vi "Lab Panel V4.83.vi"() -> ()   [LabVIEW 2013] (continued)
                    n2337 = Bundle("FAIL LAB02-2"=w3939, "SIG LAB02-2"=w3949, "TEMP START LAB02-2"=w3948, "DISP LAB02-2"=w3945, "SET LAB02-2"=w3944, "TDMS LAB02-2"=w3947) -> (w3934:T31)  [unwired: 1 in]
                    n2338 = call "sub vi - cycle&temp fail v6.vi"("Amps Lo?"=w3946, "Input Cluster"=w3934, "SELECT"=w3943, "Amps Hi?"=w3942, "Result In"=w3936) -> ("(FAIL) out"=w3938:cluster{"FAIL LO":dbl, "FAIL HI":dbl}, "(DISP) out"=w3941:T4, "T-RISE"=w3935:cluster{"T-RISE (L)":dbl, "T-RISE (N)":dbl}, "Result Out"=w3937:bool, "file error"=w3940:errorcluster)  [unwired: 10 in]
                    n2339 = local write "TEMP RISE LAB02-2"(w3935) -> ()
                    n2340 = local write "FAIL LAB02-2"(w3938) -> ()
                    n2341 = local write "DISP LAB02-2"(w3941) -> ()
                    n2342 = local write "RESULT LAB02-2"(w3937) -> ()
                    n2343 = local write "data file error"(w3940) -> ()
                  }
                }
              }
              frame #4 {
                # "LAB03-1"
                n2344 = case shown="True" w3951 {
                  tunnel: w3953 -> [_ w3966]
                  tunnel: w3950 -> [_ w3963]
                  tunnel: w3952 -> [_ w3962]
                  frame False {
                  }
                  frame True {
                    n2345 = local read "TEMP START LAB03-1"() -> (w3968:cluster{"TL":dbl, "TN":dbl})
                    n2346 = local read "FAIL LAB03-1"() -> (w3959:cluster{"LO":dbl, "HI":dbl})
                    n2347 = local read "TDMS LAB03-1"() -> (w3967:refnum<k34>)
                    n2348 = local read "SET LAB03-1"() -> (w3964:T5)
                    n2349 = local read "DISP LAB03-1"() -> (w3965:T4)
                    n2350 = local read "SIG LAB03-1"() -> (w3969:T2)
                    n2351 = local read "RESULT LAB03-1"() -> (w3956:bool)
                    n2352 = Bundle("FAIL LAB03-1"=w3959, "SIG LAB03-1"=w3969, "TEMP START LAB03-1"=w3968, "DISP LAB03-1"=w3965, "SET LAB03-1"=w3964, "TDMS LAB03-1"=w3967) -> (w3954:T32)  [unwired: 1 in]
                    n2353 = call "sub vi - cycle&temp fail v6.vi"("Amps Lo?"=w3966, "Input Cluster"=w3954, "SELECT"=w3963, "Amps Hi?"=w3962, "Result In"=w3956) -> ("(FAIL) out"=w3958:cluster{"FAIL LO":dbl, "FAIL HI":dbl}, "(DISP) out"=w3961:T4, "T-RISE"=w3955:cluster{"T-RISE (L)":dbl, "T-RISE (N)":dbl}, "Result Out"=w3957:bool, "file error"=w3960:errorcluster)  [unwired: 10 in]
                    n2354 = local write "TEMP RISE LAB03-1"(w3955) -> ()
                    n2355 = local write "FAIL LAB03-1"(w3958) -> ()
                    n2356 = local write "DISP LAB03-1"(w3961) -> ()
                    n2357 = local write "RESULT LAB03-1"(w3957) -> ()
                    n2358 = local write "data file error"(w3960) -> ()
                  }
                }
              }
              frame #5 {
                # "LAB03-2"
                n2359 = case shown="True" w3971 {
                  tunnel: w3973 -> [_ w3986]
                  tunnel: w3970 -> [_ w3983]
                  tunnel: w3972 -> [_ w3982]
                  frame False {
                  }
                  frame True {
                    n2360 = local read "TEMP START LAB03-2"() -> (w3988:cluster{"TL":dbl, "TN":dbl})
                    n2361 = local read "FAIL LAB03-2"() -> (w3979:cluster{"LO":dbl, "HI":dbl})
                    n2362 = local read "TDMS LAB03-2"() -> (w3987:refnum<k34>)
                    n2363 = local read "SET LAB03-2"() -> (w3984:T5)
                    n2364 = local read "DISP LAB03-2"() -> (w3985:T4)
                    n2365 = local read "RESULT LAB03-2"() -> (w3976:bool)
                    n2366 = local read "SIG LAB03-2"() -> (w3989:T2)
                    n2367 = Bundle("FAIL LAB03-2"=w3979, "SIG LAB03-2"=w3989, "TEMP START LAB03-2"=w3988, "DISP LAB03-2"=w3985, "SET LAB03-2"=w3984, "TDMS LAB03-2"=w3987) -> (w3974:T33)  [unwired: 1 in]
                    n2368 = call "sub vi - cycle&temp fail v6.vi"("Amps Lo?"=w3986, "Input Cluster"=w3974, "SELECT"=w3983, "Amps Hi?"=w3982, "Result In"=w3976) -> ("(FAIL) out"=w3978:cluster{"FAIL LO":dbl, "FAIL HI":dbl}, "(DISP) out"=w3981:T4, "T-RISE"=w3975:cluster{"T-RISE (L)":dbl, "T-RISE (N)":dbl}, "Result Out"=w3977:bool, "file error"=w3980:errorcluster)  [unwired: 10 in]
                    n2369 = local write "FAIL LAB03-2"(w3978) -> ()
                    n2370 = local write "TEMP RISE LAB03-2"(w3975) -> ()
                    n2371 = local write "DISP LAB03-2"(w3981) -> ()
                    n2372 = local write "RESULT LAB03-2"(w3977) -> ()
                    n2373 = local write "data file error"(w3980) -> ()
                  }
                }
              }
              frame #6 {
                # "LAB04-1"
                n2374 = case shown="True" w3991 {
                  tunnel: w3993 -> [_ w4006]
                  tunnel: w3990 -> [_ w4003]
                  tunnel: w3992 -> [_ w4002]
                  frame False {
                  }
                  frame True {
                    n2375 = local read "TEMP START LAB04-1"() -> (w4008:cluster{"TL":dbl, "TN":dbl})
                    n2376 = local read "FAIL LAB04-1"() -> (w3999:cluster{"LO":dbl, "HI":dbl})
                    n2377 = local read "TDMS LAB04-1"() -> (w4007:refnum<k34>)
                    n2378 = local read "SET LAB04-1"() -> (w4004:T5)
                    n2379 = local read "DISP LAB04-1"() -> (w4005:T4)
                    n2380 = local read "SIG LAB04-1"() -> (w4009:T2)
                    n2381 = local read "RESULT LAB04-1"() -> (w3996:bool)
                    n2382 = Bundle("FAIL LAB04-1"=w3999, "SIG LAB04-1"=w4009, "TEMP START LAB04-1"=w4008, "DISP LAB04-1"=w4005, "SET LAB04-1"=w4004, "TDMS LAB04-1"=w4007) -> (w3994:T34)  [unwired: 1 in]
                    n2383 = call "sub vi - cycle&temp fail v6.vi"("Amps Lo?"=w4006, "Input Cluster"=w3994, "SELECT"=w4003, "Amps Hi?"=w4002, "Result In"=w3996) -> ("(FAIL) out"=w3998:cluster{"FAIL LO":dbl, "FAIL HI":dbl}, "(DISP) out"=w4001:T4, "T-RISE"=w3995:cluster{"T-RISE (L)":dbl, "T-RISE (N)":dbl}, "Result Out"=w3997:bool, "file error"=w4000:errorcluster)  [unwired: 10 in]
                    n2384 = local write "TEMP RISE LAB04-1"(w3995) -> ()
                    n2385 = local write "FAIL LAB04-1"(w3998) -> ()
                    n2386 = local write "DISP LAB04-1"(w4001) -> ()
                    n2387 = local write "RESULT LAB04-1"(w3997) -> ()
                    n2388 = local write "data file error"(w4000) -> ()
                  }
                }
              }
              frame #7 {
                # "LAB04-2"
                n2389 = case shown="True" w4011 {
                  tunnel: w4013 -> [_ w4026]
                  tunnel: w4010 -> [_ w4023]
                  tunnel: w4012 -> [_ w4022]
                  frame False {
                  }
                  frame True {
                    n2390 = local read "TEMP START LAB04-2"() -> (w4028:cluster{"TL":dbl, "TN":dbl})
                    n2391 = local read "FAIL LAB04-2"() -> (w4019:cluster{"LO":dbl, "HI":dbl})
                    n2392 = local read "TDMS LAB04-2"() -> (w4027:refnum<k34>)
                    n2393 = local read "SET LAB04-2"() -> (w4024:T5)
                    n2394 = local read "DISP LAB04-2"() -> (w4025:T4)
                    n2395 = local read "SIG LAB04-2"() -> (w4029:T2)
                    n2396 = local read "RESULT LAB04-2"() -> (w4016:bool)
                    n2397 = Bundle("FAIL LAB04-2"=w4019, "SIG LAB04-2"=w4029, "TEMP START LAB04-2"=w4028, "DISP LAB04-2"=w4025, "SET LAB04-2"=w4024, "TDMS LAB04-2"=w4027) -> (w4014:T35)  [unwired: 1 in]
                    n2398 = call "sub vi - cycle&temp fail v6.vi"("Amps Lo?"=w4026, "Input Cluster"=w4014, "SELECT"=w4023, "Amps Hi?"=w4022, "Result In"=w4016) -> ("(FAIL) out"=w4018:cluster{"FAIL LO":dbl, "FAIL HI":dbl}, "(DISP) out"=w4021:T4, "T-RISE"=w4015:cluster{"T-RISE (L)":dbl, "T-RISE (N)":dbl}, "Result Out"=w4017:bool, "file error"=w4020:errorcluster)  [unwired: 10 in]
                    n2399 = local write "TEMP RISE LAB04-2"(w4015) -> ()
                    n2400 = local write "FAIL LAB04-2"(w4018) -> ()
                    n2401 = local write "DISP LAB04-2"(w4021) -> ()
                    n2402 = local write "RESULT LAB04-2"(w4017) -> ()
                    n2403 = local write "data file error"(w4020) -> ()
                  }
                }
              }
              frame #8 {
                # "LAB05-1"
                n2404 = case shown="True" w4031 {
                  tunnel: w4033 -> [_ w4046]
                  tunnel: w4030 -> [_ w4043]
                  tunnel: w4032 -> [_ w4042]
                  frame False {
                  }
                  frame True {
                    n2405 = local read "TEMP START LAB05-1"() -> (w4048:cluster{"TL":dbl, "TN":dbl})
                    n2406 = local read "FAIL LAB05-1"() -> (w4039:cluster{"LO":dbl, "HI":dbl})
                    n2407 = local read "TDMS LAB05-1"() -> (w4047:refnum<k34>)
                    n2408 = local read "SET LAB05-1"() -> (w4044:T5)
                    n2409 = local read "DISP LAB05-1"() -> (w4045:T4)
                    n2410 = local read "SIG LAB05-1"() -> (w4049:T2)
                    n2411 = local read "RESULT LAB05-1"() -> (w4036:bool)
                    n2412 = Bundle("FAIL LAB05-1"=w4039, "SIG LAB05-1"=w4049, "TEMP START LAB05-1"=w4048, "DISP LAB05-1"=w4045, "SET LAB05-1"=w4044, "TDMS LAB05-1"=w4047) -> (w4034:T36)  [unwired: 1 in]
                    n2413 = call "sub vi - cycle&temp fail v6.vi"("Amps Lo?"=w4046, "Input Cluster"=w4034, "SELECT"=w4043, "Amps Hi?"=w4042, "Result In"=w4036) -> ("(FAIL) out"=w4038:cluster{"FAIL LO":dbl, "FAIL HI":dbl}, "(DISP) out"=w4041:T4, "T-RISE"=w4035:cluster{"T-RISE (L)":dbl, "T-RISE (N)":dbl}, "Result Out"=w4037:bool, "file error"=w4040:errorcluster)  [unwired: 10 in]
                    n2414 = local write "TEMP RISE LAB05-1"(w4035) -> ()
                    n2415 = local write "FAIL LAB05-1"(w4038) -> ()
                    n2416 = local write "DISP LAB05-1"(w4041) -> ()
                    n2417 = local write "RESULT LAB05-1"(w4037) -> ()
                    n2418 = local write "data file error"(w4040) -> ()
                  }
                }
              }
              frame #9 {
                # "LAB05-2"
                n2419 = case shown="True" w4051 {
                  tunnel: w4053 -> [_ w4066]
                  tunnel: w4050 -> [_ w4063]
                  tunnel: w4052 -> [_ w4062]
                  frame False {
                  }
                  frame True {
                    n2420 = local read "TEMP START LAB05-2"() -> (w4068:cluster{"TL":dbl, "TN":dbl})
                    n2421 = local read "FAIL LAB05-2"() -> (w4059:cluster{"LO":dbl, "HI":dbl})
                    n2422 = local read "TDMS LAB05-2"() -> (w4067:refnum<k34>)
                    n2423 = local read "SET LAB05-2"() -> (w4064:T5)
                    n2424 = local read "DISP LAB05-2"() -> (w4065:T4)
                    n2425 = local read "SIG LAB05-2"() -> (w4069:T2)
                    n2426 = local read "RESULT LAB05-2"() -> (w4056:bool)
                    n2427 = Bundle("FAIL LAB05-2"=w4059, "SIG LAB05-2"=w4069, "TEMP START LAB05-2"=w4068, "DISP LAB05-2"=w4065, "SET LAB05-2"=w4064, "TDMS LAB05-2"=w4067) -> (w4054:T37)  [unwired: 1 in]
                    n2428 = call "sub vi - cycle&temp fail v6.vi"("Amps Lo?"=w4066, "Input Cluster"=w4054, "SELECT"=w4063, "Amps Hi?"=w4062, "Result In"=w4056) -> ("(FAIL) out"=w4058:cluster{"FAIL LO":dbl, "FAIL HI":dbl}, "(DISP) out"=w4061:T4, "T-RISE"=w4055:cluster{"T-RISE (L)":dbl, "T-RISE (N)":dbl}, "Result Out"=w4057:bool, "file error"=w4060:errorcluster)  [unwired: 10 in]
                    n2429 = local write "TEMP RISE LAB05-2"(w4055) -> ()
                    n2430 = local write "FAIL LAB05-2"(w4058) -> ()
                    n2431 = local write "DISP LAB05-2"(w4061) -> ()
                    n2432 = local write "RESULT LAB05-2"(w4057) -> ()
                    n2433 = local write "data file error"(w4060) -> ()
                  }
                }
              }
            }
          }
          frame #15 {
            # "run calibration routine"
            n2434 = local read "SET (cal)"() -> (w4070:bool)
            n2435 = case shown="True" w4070 {
              frame False {
              }
              frame True {
                n2436 = stacked-sequence {
                  seq-local: [w4071 _ _] -> [_ w4073 _]
                  frame #0 {
                    n2437 = call "CALIBRATION PASSWORD"() -> ("PASSWORD"=w4071:string)  [unwired: 17 in, 2 out]
                  }
                  frame #1 {
                    n2438 = Equal?(x=w4073, y="7777") -> (x = y?=w4072:bool)
                    n2439 = case shown="True" w4072 {
                      frame False {
                      }
                      frame True {
                        n2440 = stacked-sequence {
                          frame #0 {
                            n2441 = call "sub vi - calibration v1.vi"() -> ()  [unwired: 12 in]
                          }
                          frame #1 {
                            n2442 = call "sub vi - get calibration values v1.vi"() -> ("LAB01 (CAL)"=w4079:T12, "LAB02 (CAL)"=w4078:T13, "LAB03 (CAL)"=w4077:T12, "LAB04 (CAL)"=w4076:T12, "calibration file error out"=w4080:errorcluster, "LAB05 (CAL)"=w4075:T12)  [unwired: 10 in]
                            n2443 = local write "cal file error out"(w4080) -> ()
                            n2444 = local write "CAL LAB04"(w4076) -> ()
                            n2445 = local write "CAL LAB05"(w4075) -> ()
                            n2446 = local write "CAL LAB01"(w4079) -> ()
                            n2447 = local write "CAL LAB02"(w4078) -> ()
                            n2448 = local write "CAL LAB03"(w4077) -> ()
                          }
                        }
                      }
                    }
                  }
                  frame #2 {
                    n2449 = local write "SET (cal)"(FALSE) -> ()
                  }
                }
              }
            }
          }
          frame #16 {
            # "save certain settings to file"
            n2450 = String To Path(string="c:\\crabtree\\Set Up\\") -> (path=w4083:path)
            n2451 = Build Path(base path=w4083, name or relative path="settings.bin") -> (appended path=w4085:path)
            n2452 = Build Path(base path=w4083, name or relative path="mail.bin") -> (appended path=w4082:path)
            n2453 = Create Folder(path (use dialog)=w4083) -> (error out=w4088:errorcluster)  [unwired: 2 in, 2 out]
            n2454 = call <vilib>:"Clear Errors.vi"("error in (no error)"=w4088) -> ()  [unwired: 6 in, 1 out]
            n2455 = stacked-sequence {
              seq-local: [w4098 _] -> [_ w4111]
              tunnel: w4085 -> [_ w4112]
              tunnel: w4082 -> [_ w4110]
              frame #0 {
                n2456 = local read "C drive data root dir"() -> (w4097:path)
                n2457 = local read "Select COM port"() -> (w4094:refnum<visa-resource-name>)
                n2458 = local read "Network Directory"() -> (w4103:path)
                n2459 = local read "SET LAB05-2"() -> (w4102:T5)
                n2460 = local read "SET LAB05-1"() -> (w4101:T5)
                n2461 = local read "SET LAB04-2"() -> (w4100:T5)
                n2462 = local read "SET LAB03-2"() -> (w4104:T5)
                n2463 = local read "SET LAB04-1"() -> (w4099:T5)
                n2464 = local read "SET LAB03-1"() -> (w4105:T5)
                n2465 = local read "SET LAB02-2"() -> (w4106:T5)
                n2466 = local read "SET LAB02-1"() -> (w4107:T5)
                n2467 = local read "Temp Delay Lps"() -> (w4093:dbl)
                n2468 = local read "SET LAB01-2"() -> (w4108:T5)
                n2469 = local read "Temp Test Cal"() -> (w4090:dbl)
                n2470 = local read "SET LAB01-1"() -> (w4109:T5)
                n2471 = local read "Temp Value"() -> (w4092:dbl)
                n2472 = local read "Fail Loops"() -> (w4091:dbl)
                n2473 = local read "spare"() -> (w4089:dbl)
                n2474 = local read "RATE (Hz)"() -> (w4096:dbl)
                n2475 = local read "SAMPLES"() -> (w4095:dbl)
                n2476 = Bundle("SET LAB01-1"=w4109, "SET LAB01-2"=w4108, "SET LAB02-1"=w4107, "SET LAB02-2"=w4106, "SET LAB03-1"=w4105, "SET LAB03-2"=w4104, "SET LAB04-1"=w4099, "SET LAB04-2"=w4100, "SET LAB05-1"=w4101, "SET LAB05-2"=w4102, "Network Directory"=w4103, "C drive data root dir"=w4097, "RATE (Hz)"=w4096, "SAMPLES"=w4095, "Select COM port"=w4094, "Temp Delay Lps"=w4093, "Temp Value"=w4092, "Fail Loops"=w4091, "Temp Test Cal"=w4090, "spare"=w4089) -> (w4098:T20)  [unwired: 1 in]
              }
              frame #1 {
                n2477 = event shown="[1] \"SET LAB01-1\", \"SET LAB01-2\", \"SET LAB02-1\", \"SET LAB02-2\", \"SET LAB03-1\", \"SET LAB03-2\", \"SET LAB04-1\", \"SET LAB04-2\", \"SET LAB05-1\", \"SET LAB05-2\", \"Network Directory\", \"C drive data root dir\", \"RATE (Hz)\", \"SAMPLES\", \"Select COM port\", \"Temp Delay Lps\", \"Temp Value\", \"Fail Loops\", \"Temp Test Cal\", \"spare\": Value Change" {
                  selector: _ -> [_ _ _]
                  dyn-events: _ -> [_ _ _]
                  timeout: 10.0 -> [_ _ _]
                  tunnel: w4112 -> [_ w4114 _]
                  tunnel: w4111 -> [_ w4115 _]
                  tunnel: w4110 -> [_ _ w4126]
                  event Timeout {
                    n2478 = event-data() -> ()  [unwired: 1 in, 3 out]
                  }
                  event "SET LAB01-1", "SET LAB01-2", "SET LAB02-1", "SET LAB02-2", "SET LAB03-1", "SET LAB03-2", "SET LAB04-1", "SET LAB04-2", "SET LAB05-1", "SET LAB05-2", "Network Directory", "C drive data root dir", "RATE (Hz)", "SAMPLES", "Select COM port", "Temp Delay Lps", "Temp Value", "Fail Loops", "Temp Test Cal", "spare": Value Change {
                    n2479 = event-data() -> ()  [unwired: 1 in, 6 out]
                    n2480 = Open/Create/Replace File(file path (use dialog)=w4114, operation (0:open)=T19."replace or create") -> (refnum out=w4120:refnum<file>, error out=w4119:errorcluster)  [unwired: 4 in, 1 out]
                    n2481 = Write to Binary File(file (use dialog)=w4120, data=w4115, error in=w4119) -> (refnum out=w4118:refnum<file>, error out=w4117:errorcluster)  [unwired: 3 in, 1 out]
                    n2482 = Close File(refnum=w4118, error in=w4117) -> (error out=w4116:errorcluster)  [unwired: 1 out]
                    n2483 = local write "data file error"(w4116) -> ()
                  }
                  event "MAIL SETTINGS.OUT SERVER ADDRESS", "MAIL SETTINGS.FROM ACCOUNT", "MAIL SETTINGS.USER NAME", "MAIL SETTINGS.PASSWORD", "Auto Mail Send", "TO (string):": Value Change {
                    n2484 = event-data() -> ()  [unwired: 1 in, 6 out]
                    n2485 = local read "MAIL SETTINGS"() -> (w4125:T6)
                    n2486 = local read "Auto Mail Send"() -> (w4123:bool)
                    n2487 = local read "TO (string):"() -> (w4122:string)
                    n2488 = Open/Create/Replace File(file path (use dialog)=w4126, operation (0:open)=T19."replace or create") -> (refnum out=w4131:refnum<file>, error out=w4130:errorcluster)  [unwired: 4 in, 1 out]
                    n2489 = Bundle("MAIL SETTINGS"=w4125, "Auto Mail Send"=w4123, "TO (string):"=w4122) -> (w4124:T38)  [unwired: 1 in]
                    n2490 = Write to Binary File(file (use dialog)=w4131, data=w4124, error in=w4130) -> (refnum out=w4129:refnum<file>, error out=w4128:errorcluster)  [unwired: 3 in, 1 out]
                    n2491 = Close File(refnum=w4129, error in=w4128) -> (error out=w4127:errorcluster)  [unwired: 1 out]
                    n2492 = local write "data file error"(w4127) -> ()
                  }
                }
              }
            }
          }
          frame #17 {
            # "mail control"
            n2493 = local read "MAIL SETTINGS"() -> (w4148:T6)
            n2494 = local read "Auto Mail Send"() -> (w4134:bool)
            n2495 = Unbundle(w4148) -> ("OUT SERVER ADDRESS"=w4147:string, "FROM ACCOUNT"=w4146:string, "TEST MAIL"=w4145:bool)  [unwired: 4 out]
            n2496 = stacked-sequence {
              tunnel: "TO (string):" -> [_ w4187]
              tunnel: w4148 -> [w4153 w4186]
              tunnel: w4147 -> [w4152 w4185]
              tunnel: w4146 -> [w4151 w4184]
              tunnel: w4145 -> [w4150 _]
              tunnel: w4134 -> [_ w4183]
              tunnel: w4144 -> [_ w4182]
              tunnel: w4143 -> [_ w4181]
              tunnel: w4142 -> [_ w4180]
              tunnel: w4141 -> [_ w4179]
              tunnel: w4140 -> [_ w4178]
              tunnel: w4139 -> [_ w4177]
              tunnel: w4138 -> [_ w4176]
              tunnel: w4137 -> [_ w4175]
              tunnel: w4136 -> [_ w4174]
              tunnel: w4135 -> [_ w4173]
              tunnel: "TO (string):" -> [w4149 _]
              frame #0 {
                # "mail test"
                n2497 = case shown="True" w4150 {
                  tunnel: w4153 -> [_ w4157]
                  tunnel: w4149 -> [_ w4156]
                  tunnel: w4152 -> [_ w4155]
                  tunnel: w4151 -> [_ w4154]
                  frame False {
                  }
                  frame True {
                    n2498 = stacked-sequence {
                      seq-local: [_ _ w4167 _] -> [_ _ _ w4168]
                      tunnel: w4157 -> [w4160 _ _ w4172]
                      tunnel: w4156 -> [_ _ w4165 _]
                      tunnel: w4155 -> [_ _ w4163 _]
                      tunnel: w4154 -> [_ _ w4164 _]
                      frame #0 {
                        n2499 = Bundle(cluster=w4160, "TEST MAIL STATUS"="TEST START") -> (w4158:T6)  [unwired: 6 in]
                        n2500 = local write "MAIL SETTINGS"(w4158) -> ()
                      }
                      frame #1 {
                        n2501 = Wait (ms)(milliseconds to wait=500) -> ()  [unwired: 1 out]
                      }
                      frame #2 {
                        n2502 = call "sub vi - send mail with attach v5.vi"("TO:"=w4165, "subject"="MAIL TEST FROM LAB PANEL", "from"=w4164, "out going server"=w4163, "message"="TEST MESSAGE") -> ("error out"=w4167:errorcluster)  [unwired: 10 in]
                      }
                      frame #3 {
                        n2503 = Bundle(cluster=w4172, "TEST MAIL"=FALSE, "TEST MAIL STATUS"="TEST END", "mail error"=w4168) -> (w4170:T6)  [unwired: 4 in]
                        n2504 = local write "MAIL SETTINGS"(w4170) -> ()
                      }
                    }
                  }
                }
              }
              frame #1 {
                # "mail report"
                n2505 = stacked-sequence {
                  seq-local: [_ w4230 _ _] -> [_ _ _ w4420]
                  seq-local: [_ _ w4333 _] -> [_ _ _ w4410]
                  seq-local: [w4197 _ _ _] -> [_ w4247 _ _]
                  seq-local: [w4196 _ _ _] -> [_ w4246 _ _]
                  seq-local: [w4194 _ _ _] -> [_ w4244 _ _]
                  seq-local: [w4195 _ _ _] -> [_ w4245 _ _]
                  seq-local: [w4193 _ _ _] -> [_ w4243 _ _]
                  seq-local: [w4192 _ _ _] -> [_ w4238 _ _]
                  seq-local: [w4191 _ _ _] -> [_ w4239 _ _]
                  seq-local: [w4190 _ _ _] -> [_ w4240 _ _]
                  seq-local: [w4189 _ _ _] -> [_ w4241 _ _]
                  seq-local: [w4188 _ _ _] -> [_ w4242 _ _]
                  tunnel: w4187 -> [_ _ _ w4421]
                  tunnel: w4186 -> [_ _ _ w4404]
                  tunnel: w4185 -> [_ _ _ w4418]
                  tunnel: w4184 -> [_ _ _ w4417]
                  tunnel: w4183 -> [w4228 _ _ w4412]
                  tunnel: w4182 -> [_ _ w4363 _]
                  tunnel: w4181 -> [_ _ w4360 _]
                  tunnel: w4180 -> [_ _ w4359 _]
                  tunnel: w4179 -> [_ _ w4358 _]
                  tunnel: w4178 -> [_ _ w4357 _]
                  tunnel: w4177 -> [_ _ w4356 _]
                  tunnel: w4176 -> [_ _ w4355 _]
                  tunnel: w4175 -> [_ _ w4354 _]
                  tunnel: w4174 -> [_ _ w4353 _]
                  tunnel: w4173 -> [_ _ w4352 _]
                  frame #0 {
                    n2506 = case shown="False" w4228 {
                      frame False {
                        n2507 = local write "mail control"("") -> ()
                      }
                      frame True {
                      }
                    }
                    n2508 = local read "SET LAB01-1"() -> (w4227:T5)
                    n2509 = local read "SET LAB01-2"() -> (w4226:T5)
                    n2510 = local read "SET LAB02-1"() -> (w4225:T5)
                    n2511 = local read "SET LAB02-2"() -> (w4224:T5)
                    n2512 = local read "SET LAB03-1"() -> (w4223:T5)
                    n2513 = local read "SET LAB04-1"() -> (w4221:T5)
                    n2514 = local read "SET LAB05-1"() -> (w4219:T5)
                    n2515 = local read "SET LAB03-2"() -> (w4222:T5)
                    n2516 = local read "SET LAB04-2"() -> (w4220:T5)
                    n2517 = local read "SET LAB05-2"() -> (w4218:T5)
                    n2518 = Unbundle(w4223) -> ("DESCRIPTION"=w4203:string)  [unwired: 4 out]
                    n2519 = Unbundle(w4222) -> ("DESCRIPTION"=w4202:string)  [unwired: 4 out]
                    n2520 = Unbundle(w4221) -> ("DESCRIPTION"=w4201:string)  [unwired: 4 out]
                    n2521 = Unbundle(w4218) -> ("DESCRIPTION"=w4198:string)  [unwired: 4 out]
                    n2522 = Unbundle(w4224) -> ("DESCRIPTION"=w4204:string)  [unwired: 4 out]
                    n2523 = Unbundle(w4220) -> ("DESCRIPTION"=w4200:string)  [unwired: 4 out]
                    n2524 = Unbundle(w4227) -> ("DESCRIPTION"=w4216:string)  [unwired: 4 out]
                    n2525 = Unbundle(w4225) -> ("DESCRIPTION"=w4205:string)  [unwired: 4 out]
                    n2526 = Unbundle(w4219) -> ("DESCRIPTION"=w4199:string)  [unwired: 4 out]
                    n2527 = Unbundle(w4226) -> ("DESCRIPTION"=w4206:string)  [unwired: 4 out]
                    n2528 = Concatenate Strings("[LAB05-2/", w4198) -> (w4188:string)
                    n2529 = Concatenate Strings("[LAB05-1/", w4199) -> (w4189:string)
                    n2530 = Concatenate Strings("[LAB04-2/", w4200) -> (w4190:string)
                    n2531 = Concatenate Strings("[LAB03-2/", w4202) -> (w4192:string)
                    n2532 = Concatenate Strings("[LAB04-1/", w4201) -> (w4191:string)
                    n2533 = Concatenate Strings("[LAB03-1/", w4203) -> (w4193:string)
                    n2534 = Concatenate Strings("[LAB01-2/", w4206) -> (w4196:string)
                    n2535 = Concatenate Strings("[LAB02-2/", w4204) -> (w4194:string)
                    n2536 = Concatenate Strings("[LAB01-1/", w4216) -> (w4197:string)
                    n2537 = Concatenate Strings("[LAB02-1/", w4205) -> (w4195:string)
                  }
                  frame #1 {
                    w4251 = "/"
                    w4252 = 2.0
                    n2538 = local read "DISP LAB01-2"() -> (w4331:T4)
                    n2539 = local read "DISP LAB01-1"() -> (w4332:T4)
                    n2540 = local read "DISP LAB02-1"() -> (w4330:T4)
                    n2541 = local read "DISP LAB03-2"() -> (w4327:T4)
                    n2542 = local read "DISP LAB02-2"() -> (w4329:T4)
                    n2543 = local read "DISP LAB03-1"() -> (w4328:T4)
                    n2544 = local read "DISP LAB04-2"() -> (w4325:T4)
                    n2545 = local read "DISP LAB04-1"() -> (w4326:T4)
                    n2546 = local read "DISP LAB05-1"() -> (w4324:T4)
                    n2547 = local read "DISP LAB05-2"() -> (w4323:T4)
                    n2548 = Unbundle(w4331) -> ("CYCLE"=w4315:dbl, "MINS"=w4314:dbl, "STATUS"=w4311:string)
                    n2549 = Unbundle(w4332) -> ("CYCLE"=w4320:dbl, "MINS"=w4319:dbl, "STATUS"=w4316:string)
                    n2550 = Unbundle(w4330) -> ("CYCLE"=w4308:dbl, "MINS"=w4307:dbl, "STATUS"=w4306:string)
                    n2551 = Unbundle(w4327) -> ("CYCLE"=w4295:dbl, "MINS"=w4294:dbl, "STATUS"=w4291:string)
                    n2552 = Unbundle(w4328) -> ("CYCLE"=w4300:dbl, "MINS"=w4299:dbl, "STATUS"=w4296:string)
                    n2553 = Unbundle(w4329) -> ("CYCLE"=w4305:dbl, "MINS"=w4304:dbl, "STATUS"=w4301:string)
                    n2554 = Unbundle(w4326) -> ("CYCLE"=w4290:dbl, "MINS"=w4289:dbl, "STATUS"=w4286:string)
                    n2555 = Unbundle(w4325) -> ("CYCLE"=w4285:dbl, "MINS"=w4284:dbl, "STATUS"=w4281:string)
                    n2556 = Unbundle(w4324) -> ("CYCLE"=w4280:dbl, "MINS"=w4279:dbl, "STATUS"=w4276:string)
                    n2557 = Unbundle(w4323) -> ("CYCLE"=w4322:dbl, "MINS"=w4321:dbl, "STATUS"=w4273:string)
                    n2558 = Number To Decimal String(number=w4308) -> (decimal integer string=w4310:string)  [unwired: 1 in]
                    n2559 = Number To Decimal String(number=w4305) -> (decimal integer string=w4303:string)  [unwired: 1 in]
                    n2560 = Number To Decimal String(number=w4300) -> (decimal integer string=w4298:string)  [unwired: 1 in]
                    n2561 = Number To Decimal String(number=w4315) -> (decimal integer string=w4313:string)  [unwired: 1 in]
                    n2562 = Number To Decimal String(number=w4295) -> (decimal integer string=w4293:string)  [unwired: 1 in]
                    n2563 = Number To Decimal String(number=w4320) -> (decimal integer string=w4318:string)  [unwired: 1 in]
                    n2564 = Number To Decimal String(number=w4322) -> (decimal integer string=w4275:string)  [unwired: 1 in]
                    n2565 = Number To Decimal String(number=w4290) -> (decimal integer string=w4288:string)  [unwired: 1 in]
                    n2566 = Number To Decimal String(number=w4285) -> (decimal integer string=w4283:string)  [unwired: 1 in]
                    n2567 = Number To Decimal String(number=w4280) -> (decimal integer string=w4278:string)  [unwired: 1 in]
                    n2568 = Number To Fractional String(number=w4307, precision (6)=w4252) -> (F-format string=w4309:string)  [unwired: 2 in]
                    n2569 = Number To Fractional String(number=w4294, precision (6)=w4252) -> (F-format string=w4292:string)  [unwired: 2 in]
                    n2570 = Number To Fractional String(number=w4304, precision (6)=w4252) -> (F-format string=w4302:string)  [unwired: 2 in]
                    n2571 = Number To Fractional String(number=w4299, precision (6)=w4252) -> (F-format string=w4297:string)  [unwired: 2 in]
                    n2572 = Number To Fractional String(number=w4284, precision (6)=w4252) -> (F-format string=w4282:string)  [unwired: 2 in]
                    n2573 = Number To Fractional String(number=w4289, precision (6)=w4252) -> (F-format string=w4287:string)  [unwired: 2 in]
                    n2574 = Number To Fractional String(number=w4314, precision (6)=w4252) -> (F-format string=w4312:string)  [unwired: 2 in]
                    n2575 = Number To Fractional String(number=w4279, precision (6)=w4252) -> (F-format string=w4277:string)  [unwired: 2 in]
                    n2576 = Number To Fractional String(number=w4319, precision (6)=w4252) -> (F-format string=w4317:string)  [unwired: 2 in]
                    n2577 = Number To Fractional String(number=w4321, precision (6)=w4252) -> (F-format string=w4274:string)  [unwired: 2 in]
                    n2578 = Concatenate Strings(w4251, w4293, w4251, w4292, w4251, w4291) -> (w4267:string)
                    n2579 = Concatenate Strings(w4251, w4288, w4251, w4287, w4251, w4286) -> (w4266:string)
                    n2580 = Concatenate Strings(w4251, w4283, w4251, w4282, w4251, w4281) -> (w4265:string)
                    n2581 = Concatenate Strings(w4251, w4278, w4251, w4277, w4251, w4276) -> (w4264:string)
                    n2582 = Concatenate Strings(w4251, w4275, w4251, w4274, w4251, w4273) -> (w4263:string)
                    n2583 = Concatenate Strings(w4251, w4318, w4251, w4317, w4251, w4316) -> (w4272:string)
                    n2584 = Concatenate Strings(w4251, w4298, w4251, w4297, w4251, w4296) -> (w4268:string)
                    n2585 = Concatenate Strings(w4251, w4313, w4251, w4312, w4251, w4311) -> (w4271:string)
                    n2586 = Concatenate Strings(w4251, w4310, w4251, w4309, w4251, w4306) -> (w4270:string)
                    n2587 = Concatenate Strings(w4251, w4303, w4251, w4302, w4251, w4301) -> (w4269:string)
                    n2588 = Concatenate Strings("]", "\r") -> (w4248:string)
                    n2589 = Concatenate Strings(w4243, w4268, w4248) -> (w4258:string)
                    n2590 = Concatenate Strings(w4245, w4270, w4248) -> (w4260:string)
                    n2591 = Concatenate Strings(w4244, w4269, w4248) -> (w4259:string)
                    n2592 = Concatenate Strings(w4240, w4265, w4248) -> (w4255:string)
                    n2593 = Concatenate Strings(w4241, w4264, w4248) -> (w4256:string)
                    n2594 = Concatenate Strings(w4239, w4266, w4248) -> (w4254:string)
                    n2595 = Concatenate Strings(w4238, w4267, w4248) -> (w4253:string)
                    n2596 = Concatenate Strings(w4242, w4263, w4248) -> (w4257:string)
                    n2597 = Concatenate Strings(w4246, w4271, w4248) -> (w4261:string)
                    n2598 = Concatenate Strings(w4247, w4272, w4248) -> (w4262:string)
                    n2599 = Concatenate Strings(w4262, w4261, w4260, w4259, w4258, w4253, w4254, w4255, w4256, w4257) -> (w4231:string)
                    n2600 = Concatenate Strings("[PANEL/", "DESC/", "CYCLES/", "MINS/", "STATUS]", "\r", w4231) -> (w4230:string)
                    "MAIL REPORT" <- w4230
                    n2601 = global write "Global display 3.vi" "log all"(w4230) -> ()
                  }
                  frame #2 {
                    w4361 = "END"
                    n2602 = local read "mail control"() -> (w4362:string)
                    n2603 = case shown="False" w4357 {
                      tunnel: w4362 -> [w4386 _]
                      tunnel: w4361 -> [w4385 _]
                      tunnel: [w4384 FALSE] -> w4347
                      frame False {
                        n2604 = Equal?(x=w4386, y=w4385) -> (x = y?=w4384:bool)
                      }
                      frame True {
                      }
                    }
                    n2605 = case shown="False" w4363 {
                      tunnel: w4362 -> [w4402 _]
                      tunnel: w4361 -> [w4401 _]
                      tunnel: [w4400 FALSE] -> w4351
                      frame False {
                        n2606 = Equal?(x=w4402, y=w4401) -> (x = y?=w4400:bool)
                      }
                      frame True {
                      }
                    }
                    n2607 = case shown="False" w4360 {
                      tunnel: w4362 -> [w4398 _]
                      tunnel: w4361 -> [w4397 _]
                      tunnel: [w4396 FALSE] -> w4350
                      frame False {
                        n2608 = Equal?(x=w4398, y=w4397) -> (x = y?=w4396:bool)
                      }
                      frame True {
                      }
                    }
                    n2609 = case shown="False" w4358 {
                      tunnel: w4362 -> [w4390 _]
                      tunnel: w4361 -> [w4389 _]
                      tunnel: [w4388 FALSE] -> w4348
                      frame False {
                        n2610 = Equal?(x=w4390, y=w4389) -> (x = y?=w4388:bool)
                      }
                      frame True {
                      }
                    }
                    n2611 = case shown="False" w4359 {
                      tunnel: w4362 -> [w4394 _]
                      tunnel: w4361 -> [w4393 _]
                      tunnel: [w4392 FALSE] -> w4349
                      frame False {
                        n2612 = Equal?(x=w4394, y=w4393) -> (x = y?=w4392:bool)
                      }
                      frame True {
                      }
                    }
                    n2613 = Or(x=w4349, y=w4348) -> (x .or. y?=w4340:bool)
                    n2614 = Or(x=w4351, y=w4350) -> (x .or. y?=w4341:bool)
                    n2615 = Or(x=w4341, y=w4340) -> (x .or. y?=w4336:bool)
                    n2616 = case shown="False" w4353 {
                      tunnel: w4362 -> [w4370 _]
                      tunnel: w4361 -> [w4369 _]
                      tunnel: [w4368 FALSE] -> w4342
                      frame False {
                        n2617 = Equal?(x=w4370, y=w4369) -> (x = y?=w4368:bool)
                      }
                      frame True {
                      }
                    }
                    n2618 = case shown="False" w4352 {
                      tunnel: w4362 -> [w4366 _]
                      tunnel: w4361 -> [w4365 _]
                      tunnel: [w4364 FALSE] -> w4346
                      frame False {
                        n2619 = Equal?(x=w4366, y=w4365) -> (x = y?=w4364:bool)
                      }
                      frame True {
                      }
                    }
                    n2620 = case shown="False" w4354 {
                      tunnel: w4362 -> [w4374 _]
                      tunnel: w4361 -> [w4373 _]
                      tunnel: [w4372 FALSE] -> w4343
                      frame False {
                        n2621 = Equal?(x=w4374, y=w4373) -> (x = y?=w4372:bool)
                      }
                      frame True {
                      }
                    }
                    n2622 = case shown="False" w4356 {
                      tunnel: w4362 -> [w4382 _]
                      tunnel: w4361 -> [w4381 _]
                      tunnel: [w4380 FALSE] -> w4345
                      frame False {
                        n2623 = Equal?(x=w4382, y=w4381) -> (x = y?=w4380:bool)
                      }
                      frame True {
                      }
                    }
                    n2624 = case shown="False" w4355 {
                      tunnel: w4362 -> [w4378 _]
                      tunnel: w4361 -> [w4377 _]
                      tunnel: [w4376 FALSE] -> w4344
                      frame False {
                        n2625 = Equal?(x=w4378, y=w4377) -> (x = y?=w4376:bool)
                      }
                      frame True {
                      }
                    }
                    n2626 = Or(x=w4345, y=w4344) -> (x .or. y?=w4339:bool)
                    n2627 = Or(x=w4343, y=w4342) -> (x .or. y?=w4338:bool)
                    n2628 = Or(x=w4346, y=w4347) -> (x .or. y?=w4334:bool)
                    n2629 = Or(x=w4339, y=w4338) -> (x .or. y?=w4337:bool)
                    n2630 = Or(x=w4336, y=w4337) -> (x .or. y?=w4335:bool)
                    n2631 = Or(x=w4335, y=w4334) -> (x .or. y?=w4333:bool)
                  }
                  frame #3 {
                    n2632 = local read "on loops"() -> (w4416:dbl)
                    n2633 = local read "jig cycle"() -> (w4413:dbl)
                    n2634 = local read "Send Mail Now"() -> (w4407:bool)
                    n2635 = Add(x=w4416, y=3.0) -> (x+y=w4414:dbl)
                    n2636 = Equal?(x=w4413, y=w4414) -> (x = y?=w4408:bool)
                    n2637 = And(x=w4408, y=w4407) -> (x .and. y?=w4406:bool)
                    n2638 = And(x=w4412, y=w4408) -> (x .and. y?=w4411:bool)
                    n2639 = And(x=w4411, y=w4410) -> (x .and. y?=w4409:bool)
                    n2640 = Or(x=w4409, y=w4406) -> (x .or. y?=w4405:bool)
                    n2641 = case shown="True" w4405 {
                      tunnel: w4421 -> [_ w4427]
                      tunnel: w4420 -> [_ w4426]
                      tunnel: "Lab Panel Test Status" -> [_ w4425]
                      tunnel: w4418 -> [_ w4424]
                      tunnel: w4417 -> [_ w4423]
                      tunnel: w4404 -> [_ w4422]
                      frame False {
                      }
                      frame True {
                        n2642 = stacked-sequence {
                          tunnel: w4427 -> [w4435 _]
                          tunnel: w4426 -> [w4434 _]
                          tunnel: w4425 -> [w4433 _]
                          tunnel: w4424 -> [w4432 _]
                          tunnel: w4423 -> [w4431 _]
                          tunnel: w4422 -> [w4430 _]
                          frame #0 {
                            n2643 = call "sub vi - send mail with attach v5.vi"("TO:"=w4435, "subject"=w4433, "from"=w4431, "out going server"=w4432, "message"=w4434) -> ("error out"=w4429:errorcluster)  [unwired: 10 in]
                            n2644 = Bundle(cluster=w4430, "mail error"=w4429) -> (w4428:T6)  [unwired: 6 in]
                            n2645 = local write "MAIL SETTINGS"(w4428) -> ()
                          }
                          frame #1 {
                            n2646 = local write "mail control"("") -> ()
                            n2647 = local write "Send Mail Now"(FALSE) -> ()
                          }
                        }
                      }
                    }
                  }
                }
              }
            }
          }
          frame #18 {
            # "save jig cycle values once all run switches are off"
            n2648 = stacked-sequence {
              tunnel: w4447 -> [_ w4476]
              tunnel: w4446 -> [_ w4475]
              tunnel: w4445 -> [_ w4474]
              tunnel: w4444 -> [_ w4473]
              tunnel: w4443 -> [_ w4472]
              tunnel: w4442 -> [_ w4471]
              tunnel: w4441 -> [_ w4470]
              tunnel: w4440 -> [_ w4469]
              tunnel: w4439 -> [_ w4468]
              tunnel: w4438 -> [_ w4467]
              frame #0 {
              }
              frame #1 {
                n2649 = Not(x=w4467) -> (.not. x?=w4450:bool)
                n2650 = Not(x=w4475) -> (.not. x?=w4465:bool)
                n2651 = Not(x=w4472) -> (.not. x?=w4460:bool)
                n2652 = Not(x=w4470) -> (.not. x?=w4456:bool)
                n2653 = Not(x=w4468) -> (.not. x?=w4452:bool)
                n2654 = Not(x=w4476) -> (.not. x?=w4466:bool)
                n2655 = Not(x=w4474) -> (.not. x?=w4464:bool)
                n2656 = Not(x=w4471) -> (.not. x?=w4458:bool)
                n2657 = Not(x=w4473) -> (.not. x?=w4462:bool)
                n2658 = Not(x=w4469) -> (.not. x?=w4454:bool)
                n2659 = local read "Save JC"() -> (w4478:bool)
                n2660 = And(x=w4466, y=w4465) -> (x .and. y?=w4463:bool)
                n2661 = And(x=w4463, y=w4464) -> (x .and. y?=w4461:bool)
                n2662 = And(x=w4461, y=w4462) -> (x .and. y?=w4459:bool)
                n2663 = And(x=w4459, y=w4460) -> (x .and. y?=w4457:bool)
                n2664 = And(x=w4457, y=w4458) -> (x .and. y?=w4455:bool)
                n2665 = And(x=w4455, y=w4456) -> (x .and. y?=w4453:bool)
                n2666 = And(x=w4453, y=w4454) -> (x .and. y?=w4451:bool)
                n2667 = And(x=w4451, y=w4452) -> (x .and. y?=w4449:bool)
                n2668 = And(x=w4449, y=w4450) -> (x .and. y?=w4448:bool)
                n2669 = And(x=w4448, y=w4478) -> (x .and. y?=w4477:bool)
                n2670 = case shown="True" w4477 {
                  tunnel: w4448 -> [w4479 _]
                  frame False {
                    n2671 = case shown="False" w4479 {
                      frame False {
                        n2672 = local write "Save JC"(TRUE) -> ()
                      }
                      frame True {
                      }
                    }
                  }
                  frame True {
                    n2673 = stacked-sequence {
                      frame #0 {
                        n2674 = String To Path(string="c:\\crabtree\\Jig Cycles\\") -> (path=w4491:path)
                        n2675 = Build Path(base path=w4491, name or relative path="jigcycles.bin") -> (appended path=w4489:path)
                        n2676 = Create Folder(path (use dialog)=w4491) -> (error out=w4493:errorcluster)  [unwired: 2 in, 2 out]
                        n2677 = local read "JIG RELAY CYCLES"() -> (w4483:T7)
                        n2678 = call <vilib>:"Clear Errors.vi"("error in (no error)"=w4493) -> ()  [unwired: 6 in, 1 out]
                        n2679 = local write "Save JC"(FALSE) -> ()
                        n2680 = Open/Create/Replace File(file path (use dialog)=w4489, operation (0:open)=T19."replace or create") -> (refnum out=w4487:refnum<file>, error out=w4488:errorcluster)  [unwired: 4 in, 1 out]
                        n2681 = Write to Binary File(file (use dialog)=w4487, data=w4483, error in=w4488) -> (refnum out=w4486:refnum<file>, error out=w4485:errorcluster)  [unwired: 3 in, 1 out]
                        n2682 = Close File(refnum=w4486, error in=w4485) -> (error out=w4484:errorcluster)  [unwired: 1 out]
                        n2683 = local write "data file error"(w4484) -> ()
                      }
                      frame #1 {
                        n2684 = local read "JIG RELAY CYCLES"() -> (w4516:T7)
                        n2685 = Unbundle By Name(w4516) -> ("LAB01-1"=w4511:dbl, "LAB01-2"=w4510:dbl, "LAB02-1"=w4508:dbl, "LAB02-2"=w4507:dbl, "LAB03-1"=w4505:dbl, "LAB03-2"=w4502:dbl, "LAB04-1"=w4501:dbl, "LAB04-2"=w4499:dbl, "LAB05-1"=w4497:dbl, "LAB05-2"=w4495:dbl)
                        n2686 = stacked-sequence {
                          tunnel: w4511 -> [w4519 _ _ _ _ _ _ _ _ _]
                          tunnel: 1000000 -> [w4522 w4532 w4542 w4552 w4562 w4572 w4582 w4592 w4602 w4612]
                          tunnel: [w4520 _ _ _ _ _ _ _ _ _] -> w4514
                          tunnel: "TEST STATION HAS REACHED 1 MILLION CYCLES, REPLACE  CONTROL RELAYS" -> [w4518 w4530 w4540 w4550 w4560 w4570 w4580 w4590 w4600 w4610]
                          tunnel: [_ w4529 _ _ _ _ _ _ _ _] -> w4512
                          tunnel: w4510 -> [_ w4528 _ _ _ _ _ _ _ _]
                          tunnel: [_ _ w4539 _ _ _ _ _ _ _] -> w4509
                          tunnel: w4508 -> [_ _ w4538 _ _ _ _ _ _ _]
                          tunnel: w4507 -> [_ _ _ w4549 _ _ _ _ _ _]
                          tunnel: [_ _ _ w4548 _ _ _ _ _ _] -> w4506
                          tunnel: w4505 -> [_ _ _ _ w4559 _ _ _ _ _]
                          tunnel: [_ _ _ _ w4558 _ _ _ _ _] -> w4504
                          tunnel: [_ _ _ _ _ w4569 _ _ _ _] -> w4503
                          tunnel: w4502 -> [_ _ _ _ _ w4568 _ _ _ _]
                          tunnel: w4501 -> [_ _ _ _ _ _ w4579 _ _ _]
                          tunnel: [_ _ _ _ _ _ w4578 _ _ _] -> w4500
                          tunnel: w4499 -> [_ _ _ _ _ _ _ w4589 _ _]
                          tunnel: [_ _ _ _ _ _ _ w4588 _ _] -> w4498
                          tunnel: w4497 -> [_ _ _ _ _ _ _ _ w4599 _]
                          tunnel: [_ _ _ _ _ _ _ _ w4598 _] -> w4496
                          tunnel: w4495 -> [_ _ _ _ _ _ _ _ _ w4609]
                          tunnel: [_ _ _ _ _ _ _ _ _ w4608] -> w4494
                          frame #0 {
                            n2687 = Greater?(x=w4519, y=w4522) -> (0:w4521:bool)
                            n2688 = case shown="True" w4521 {
                              tunnel: [w4523 0] -> w4520
                              tunnel: w4519 -> [w4523 _]
                              tunnel: w4518 -> [_ w4524]
                              frame False {
                              }
                              frame True {
                                n2689 = Concatenate Strings("LA01-1 ", w4524) -> (w4527:string)
                                n2690 = One Button Dialog(message=w4527) -> ()  [unwired: 1 in, 1 out]
                              }
                            }
                          }
                          frame #1 {
                            n2691 = Greater?(x=w4528, y=w4532) -> (0:w4531:bool)
                            n2692 = case shown="True" w4531 {
                              tunnel: [w4533 0] -> w4529
                              tunnel: w4528 -> [w4533 _]
                              tunnel: w4530 -> [_ w4534]
                              frame False {
                              }
                              frame True {
                                n2693 = Concatenate Strings("LA01-2 ", w4534) -> (w4537:string)
                                n2694 = One Button Dialog(message=w4537) -> ()  [unwired: 1 in, 1 out]
                              }
                            }
                          }
                          frame #2 {
                            n2695 = Greater?(x=w4538, y=w4542) -> (0:w4541:bool)
                            n2696 = case shown="True" w4541 {
                              tunnel: [w4543 0] -> w4539
                              tunnel: w4538 -> [w4543 _]
                              tunnel: w4540 -> [_ w4544]
                              frame False {
                              }
                              frame True {
                                n2697 = Concatenate Strings("LA02-1 ", w4544) -> (w4547:string)
